vi "Setup Statically-Linked subWorkers.vi"(8 "error in":errorcluster, 11 "sequenceManagerTest in":refnum<class "sequenceManagerTest.lvclass">) -> (0 "error out":errorcluster, 3 "sequenceManagerTest out":refnum<class "sequenceManagerTest.lvclass">)   [LabVIEW 2023, in "sequenceManagerTest.lvclass"]
doc: "This VI performs a setup of all the statically-linked subWorkers that belong to the Worker that owns this VI. This VI must be called <b>before</b> any statically-linked subWorkers are called."
uses:
  sequenceManagerTest.lvclass
  sequenceManagerTest.lvclass/sequenceManagerTest.ctl
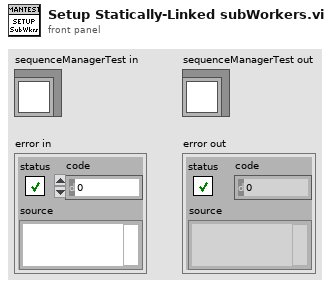
[diagram p1: front panel]
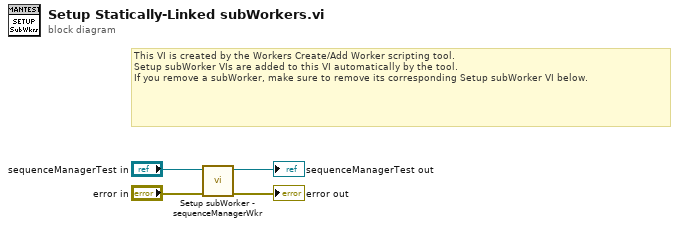
[diagram p0: block diagram]
diagram:
  # "This VI is created by the Workers Create/Add Worker scripting tool.\nSetup subWorker VIs are added to this VI automatically by the tool.\nIf you remove a subWorker, make sure to remove its corresponding Setup subWorker VI below."
  n1 = call "Setup subWorker - sequenceManagerWkr.vi"("error in"="error in", "sequenceManagerTest in"="sequenceManagerTest in") -> ("error out"=→"error out":errorcluster, "sequenceManagerTest out"=→"sequenceManagerTest out":refnum<class "sequenceManagerTest.lvclass">)  [unwired: 8 in]
